vi "Init.vi"() -> (3 "Template Msg Strategy out":refnum<class "Template Msg Strategy.lvclass">)   [LabVIEW 2021, in "_Refactor Msg.lvlib" / "jettl Msg Template.lvlib" / "Template Msg Strategy.lvclass"]
uses:
  Template Msg Strategy.lvclass
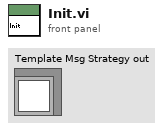
[diagram p1: front panel]
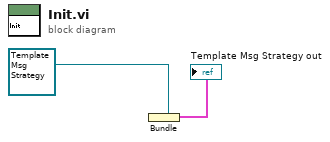
[diagram p0: block diagram]
diagram:
  n1 = Bundle "Bundle"(cluster=refnum<class "Template Msg Strategy.lvclass"> refnum ("Template Msg Strategy")) -> (→"Template Msg Strategy out":cluster{void})  [unwired: 1 in]
